vi "Ist mit Soll vergleichen UsrVal.vi"(8 "error in (no error)":errorcluster caption="Fehler (Eingang, kein Fehler)", 11 "mini8 Steuerung PNS Eingang":refnum<class "mini8 Steuerung PNS.lvclass">) -> (0 "error out":errorcluster caption="Fehler (Ausgang)", 2 "Werte":cluster{i32[], u16[]}, 3 "mini8 Steuerung PNS Ausgang":refnum<class "mini8 Steuerung PNS.lvclass">)   [LabVIEW 2020, in "mini8 Steuerung PNS.lvclass"]
uses:
  mini8 Steuerung PNS.lvclass
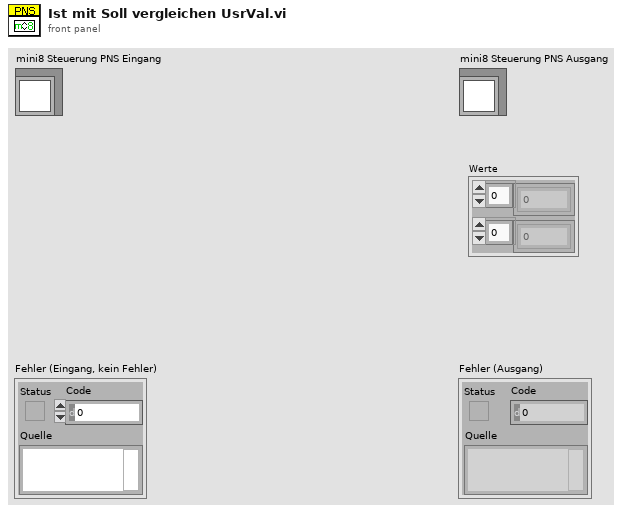
[diagram p1: front panel]
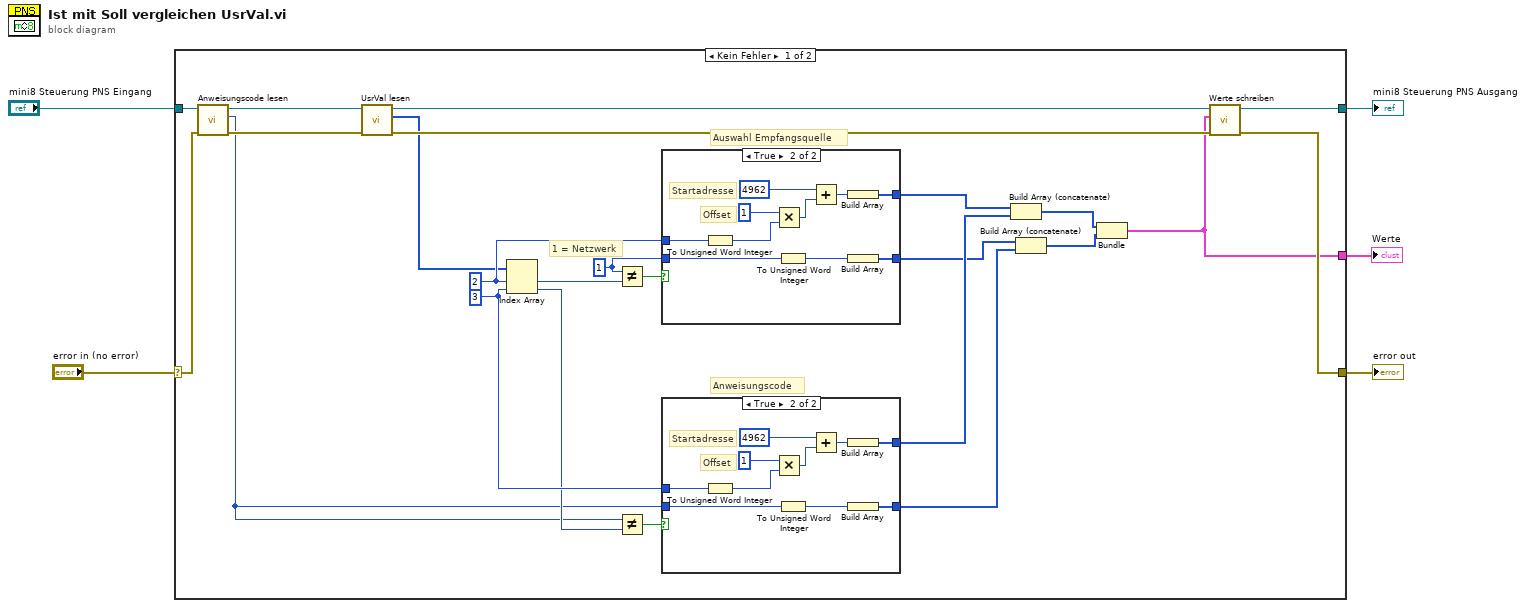
[diagram p0: block diagram]
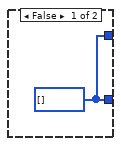
[diagram p2: hidden frame]
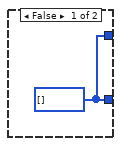
[diagram p3: hidden frame]
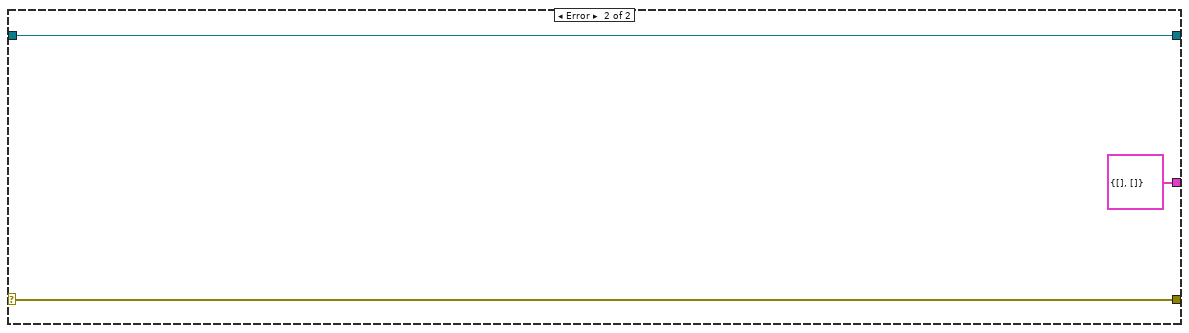
[diagram p4: hidden frame]
diagram:
  n1 = case shown="Kein Fehler" "error in (no error)" {
    selector: "error in (no error)" -> [w23 w54]
    tunnel: [w22 w54] -> w4
    tunnel: [w26 w53] -> w2
    tunnel: "mini8 Steuerung PNS Eingang" -> [w29 w53]
    tunnel: [w6 cluster{u16[], u16[]} {[], []}] -> w1
    frame No Error {
      w20 = u16 1 ("y")
      w17 = 3 ("Index")
      w11 = 2 ("Index")
      # "1 = Netzwerk"
      # "Anweisungscode"
      # "Auswahl Empfangsquelle"
      n2 = call-dynamic "Anweisungscode lesen.vi"("error in (no error)"=w23, "Steuerung PNS (Eingang)"=w29) -> ("error out"=w25:errorcluster, "Anweisungscode"=w9:u16, "Steuerung PNS (Ausgang)"=w28:refnum<class "mini8 Steuerung PNS.lvclass">)  [unwired: 7 in]
      n3 = call-dynamic "UsrVal lesen.vi"("error in (no error)"=w25, "Steuerung PNS (Eingang)"=w28) -> ("error out"=w24:errorcluster, "UsrVal"=w10:u16[], "Steuerung PNS (Ausgang)"=w27:refnum<class "mini8 Steuerung PNS.lvclass">)  [unwired: 7 in]
      n4 = Index Array(array=w10, index #1=w11, index #2=w17) -> (element #1=w19:u16, element #2=w16:u16)
      n5 = Not Equal?(x=w20, y=w19) -> (x != y?=w21:bool)
      n6 = Not Equal?(x=w9, y=w16) -> (x != y?=w18:bool)
      n7 = case shown="True" w21 {
        tunnel: w20 -> [_ w47]
        tunnel: [w41 w45] -> w15
        tunnel: [w41 w44] -> w13
        tunnel: w11 -> [_ w43]
        frame False {
          w41 = u16[] []
        }
        frame True {
          # "Offset"
          # "Startadresse"
          n8 = To Unsigned Word Integer(number=w43) -> (unsigned 16bit integer=w42:u16)
          n9 = Multiply(x=u16 1, y=w42) -> (x*y=w51:u16)
          n10 = To Unsigned Word Integer(number=w47) -> (unsigned 16bit integer=w46:u16)
          n11 = Add(x=u16 4962, y=w51) -> (x+y=w48:u16)
          n12 = Build Array(w48) -> (w45:u16[])
          n13 = Build Array(w46) -> (w44:u16[])
        }
      }
      n14 = case shown="True" w18 {
        tunnel: w9 -> [_ w36]
        tunnel: [w30 w34] -> w14
        tunnel: [w30 w33] -> w12
        tunnel: w17 -> [_ w32]
        frame False {
          w30 = u16[] []
        }
        frame True {
          # "Offset"
          # "Startadresse"
          n15 = To Unsigned Word Integer(number=w32) -> (unsigned 16bit integer=w31:u16)
          n16 = Multiply(x=u16 1, y=w31) -> (x*y=w40:u16)
          n17 = To Unsigned Word Integer(number=w36) -> (unsigned 16bit integer=w35:u16)
          n18 = Add(x=u16 4962, y=w40) -> (x+y=w37:u16)
          n19 = Build Array(w37) -> (w34:u16[])
          n20 = Build Array(w35) -> (w33:u16[])
        }
      }
      n21 = Build Array (concatenate)(w15, w14) -> (w8:u16[])
      n22 = Build Array (concatenate)(w13, w12) -> (w7:u16[])
      n23 = Bundle(w8, w7) -> (w6:cluster{u16[], u16[]})  [unwired: 1 in]
      n24 = call-dynamic "Werte schreiben.vi"("error in (no error)"=w24, "Werte"=w6, "Steuerung PNS (Eingang)"=w27) -> ("error out"=w22:errorcluster, "Steuerung PNS (Ausgang)"=w26:refnum<class "mini8 Steuerung PNS.lvclass">)  [unwired: 7 in]
    }
    frame Error {
    }
  }
  "error out" <- w4
  "mini8 Steuerung PNS Ausgang" <- w2
  "Werte" <- w1
